vi "String.Notification Message - Set Text Box State.vi"(8 "error in (no error)":errorcluster, 9 "NewColor":u32(colorbox)=16775210, 10 "Message":string, 11 "TxtBoxRef":refnum<vi>) -> (0 "error out":errorcluster, 1 "OldColor":u32(colorbox)=13816530, 2 "OldValue":string, 3 "RefOut":refnum<vi>)   [LabVIEW 2018]
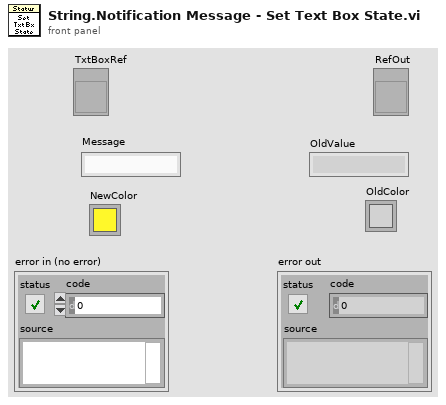
[diagram p1: front panel]
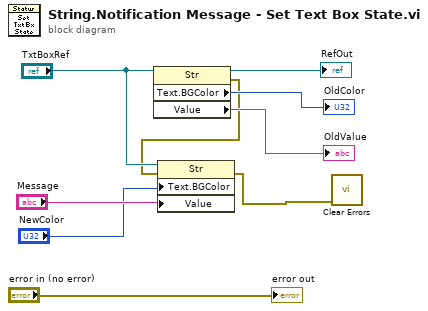
[diagram p0: block diagram]
diagram:
  n1 = property class="Str"(reference="TxtBoxRef") -> (reference out=→"RefOut":refnum<vi>, error out=w2:errorcluster, "Text.BGColor"=→"OldColor":u32, "Value"=→"OldValue":string)  [unwired: 1 in]
  n2 = property class="Str"(reference="TxtBoxRef", error in=w2, "Text.BGColor"="NewColor", "Value"="Message") -> (error out=w1:errorcluster)  [unwired: 1 out]
  n3 = call <vilib>:"Clear Errors.vi"("error in (no error)"=w1) -> ()  [unwired: 5 in, 2 out]
  "error out" <- "error in (no error)"
